vi "Engine-RPC-Plot-Host.vi"() -> ()   [LabVIEW 2016]
uses:
  Shared/Typedefs/Engine-RPC-Modes.ctl
  Shared/DSI-Shared.lvlib
panel:
  out "_Setpoint 1":sgl caption="Setpoint 1"
  out "_Setpoint2Unit":string
  out "_Sensor2Unit":string
  out "_Sensor 2":sgl caption="Sensor 2"
  out "_Setpoint 2":sgl caption="Setpoint 2"
  out "_Setpoint1Unit":string
  out "_Sensor1Unit":string
  out "_Sensor 1":sgl caption="Sensor 1"
  in  "PWM-B_RailPStp":sgl caption="[bar]"
  in  "PWM-A_RailPStp":sgl caption="[bar]"
  in  "Sync-A_RailPStp":sgl caption="[bar]"
  in  "Sync-B_RailPStp":sgl caption="[bar]"
  in  "_Control Mode":T1 caption="Control Mode"
  out "Sync-B_RailP":T2 caption="Sensor"
  out "Sync-A_RailP":T2 caption="Sensor"
  out "PWM-B_RailP":T2 caption="Sensor"
  out "PWM-A_RailP":T2 caption="Sensor"
  out "_Rail Pressure Plot":T3(graph)
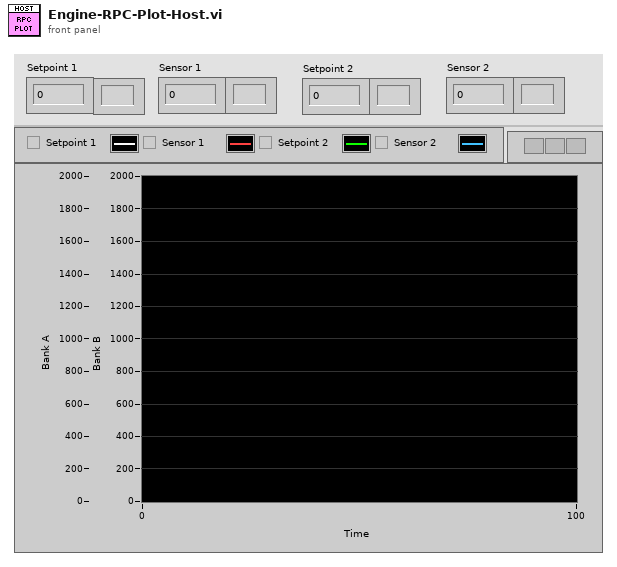
[diagram p1: front panel]
types:
  T1 = typedef "DSI-Shared.lvlib/Engine-RPC-Modes.ctl" = enum8{"Disabled", "DSI - PWM Pumps", "DSI - Sync Pumps", "User Plugin"}
  T2 = cluster{"Name":string, "Unit":string, "Value":sgl}
  T3 = cluster{"Sync-A_RailPStp":sgl, "Value":sgl, "Sync-B_RailPStp":sgl, "Value":sgl}
  T4 = cluster{"PWM-A_RailPStp":sgl, "Value":sgl, "PWM-B_RailPStp":sgl, "Value":sgl}
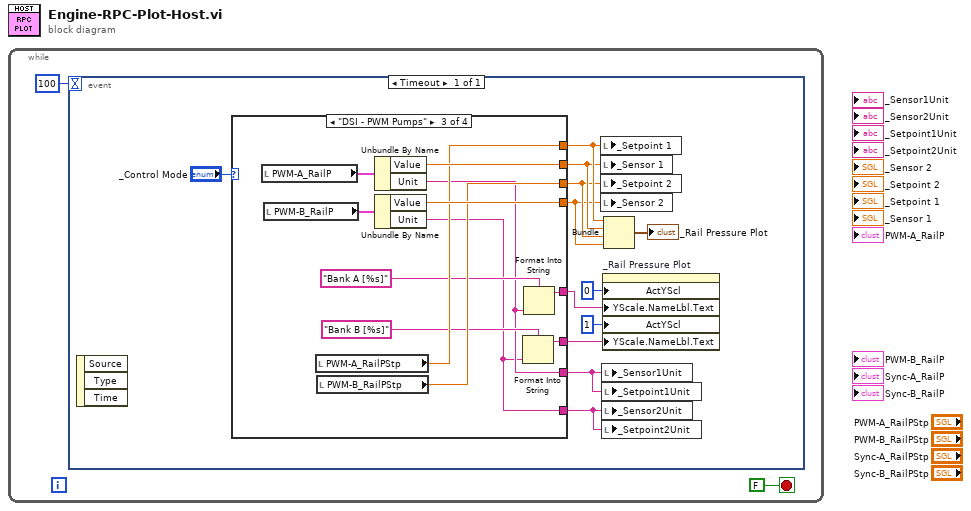
[diagram p0: block diagram]
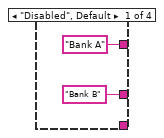
[diagram p2: hidden frame]
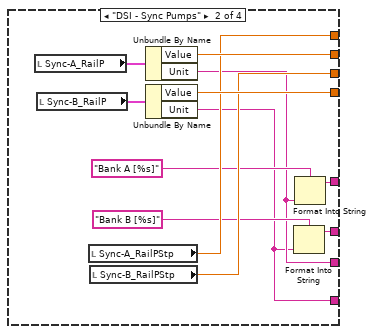
[diagram p3: hidden frame]
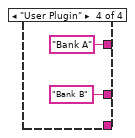
[diagram p4: hidden frame]
diagram:
  n1 = while {
    stop <- FALSE stop-if-true
    n2 = event shown="[0] Timeout" {
      selector: _ -> [_]
      dyn-events: _ -> [_]
      timeout: 100 -> [_]
      event Timeout {
        n3 = event-data() -> ()  [unwired: 1 in, 3 out]
        n4 = case shown="\"DSI - PWM Pumps\"" "_Control Mode" {
          tunnel: [_ w26 w38 _] -> w9
          tunnel: [_ w25 w37 _] -> w7
          tunnel: [_ w20 w32 _] -> w12
          tunnel: [_ w19 w31 _] -> w11
          tunnel: [_ w24 w36 _] -> w10
          tunnel: [_ w23 w35 _] -> w8
          tunnel: ["Bank B" w18 w30 "Bank B"] -> w4
          tunnel: ["Bank A" w17 w29 "Bank A"] -> w3
          frame "Disabled", Default {
          }
          frame "DSI - Sync Pumps" {
            n5 = local read "Sync-A_RailP"() -> (w28:T2)
            n6 = local read "Sync-B_RailP"() -> (w27:T2)
            n7 = local read "Sync-A_RailPStp"() -> (w24:sgl)
            n8 = local read "Sync-B_RailPStp"() -> (w23:sgl)
            n9 = Unbundle By Name(w28) -> ("Value"=w26:sgl, "Unit"=w20:string)
            n10 = Unbundle By Name(w27) -> ("Value"=w25:sgl, "Unit"=w19:string)
            n11 = Format Into String(format string="Bank B [%s]" ("Unit"), w19) -> (resulting string=w18:string)  [unwired: 2 in, 1 out]
            n12 = Format Into String(format string="Bank A [%s]" ("Unit"), w20) -> (resulting string=w17:string)  [unwired: 2 in, 1 out]
          }
          frame "DSI - PWM Pumps" {
            n13 = local read "PWM-A_RailP"() -> (w40:T2)
            n14 = local read "PWM-B_RailP"() -> (w39:T2)
            n15 = local read "PWM-A_RailPStp"() -> (w36:sgl)
            n16 = local read "PWM-B_RailPStp"() -> (w35:sgl)
            n17 = Unbundle By Name(w40) -> ("Value"=w38:sgl, "Unit"=w32:string)
            n18 = Unbundle By Name(w39) -> ("Value"=w37:sgl, "Unit"=w31:string)
            n19 = Format Into String(format string="Bank B [%s]" ("Unit"), w31) -> (resulting string=w30:string)  [unwired: 2 in, 1 out]
            n20 = Format Into String(format string="Bank A [%s]" ("Unit"), w32) -> (resulting string=w29:string)  [unwired: 2 in, 1 out]
          }
          frame "User Plugin" {
          }
        }
        n21 = local write "_Setpoint 1"(w10) -> ()
        n22 = local write "_Sensor 1"(w9) -> ()
        n23 = local write "_Setpoint 2"(w8) -> ()
        n24 = local write "_Sensor 2"(w7) -> ()
        n25 = local write "_Sensor1Unit"(w12) -> ()
        n26 = local write "_Setpoint1Unit"(w12) -> ()
        n27 = local write "_Sensor2Unit"(w11) -> ()
        n28 = local write "_Setpoint2Unit"(w11) -> ()
        n29 = property on="_Rail Pressure Plot" class="WFChart (strict)"("ActYScl"=0 ("Active Y Scale"), "YScale.NameLbl.Text"=w3, "ActYScl"=1 ("Active Y Scale"), "YScale.NameLbl.Text"=w4) -> ()  [unwired: 2 in, 2 out]
        n30 = Bundle("PWM-A_RailPStp"=w10, "Value"=w9, "PWM-B_RailPStp"=w8, "Value"=w7) -> (→"_Rail Pressure Plot":T4)  [unwired: 1 in]
      }
    }
  }
